vi "wait with error cluster.vi"(8 "error in":errorcluster, 11 "wait (ms)":u32) -> (0 "error out":errorcluster)   [LabVIEW 2020, in "Reusable Library.lvlib"]
uses:
  Reusable Library.lvlib
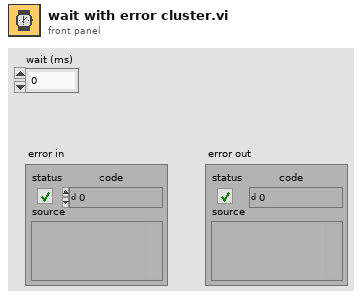
[diagram p1: front panel]
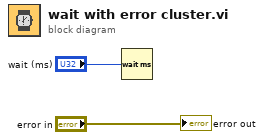
[diagram p0: block diagram]
diagram:
  n1 = Wait (ms)(milliseconds to wait="wait (ms)") -> ()  [unwired: 1 out]
  "error out" <- "error in"
